vi "写入excel(幅频响应).vi"(7 "设置":string[](array[string])=["160", "10", "0.02", "0.02", "0.1", "10", "J5", "J6"], 8 "error in (no error)":errorcluster, 9 "被测幅值":dbl format="%.2p", 10 "参考幅值":dbl format="%.2p", 11 "NI_report输入":refnum<class "NI_report.lvclass">) -> (0 "error out":errorcluster, 3 "report out":refnum<class "NI_report.lvclass">)   [LabVIEW 2015]
uses:
  <vilib>/Utility/NIReport.llb/NI_report.lvclass
  <vilib>/addons/_office/_exclsub.llb/font.ctl
  Global.vi
  <vilib>/Utility/NIReport.llb/Excel/NI_Excel.lvclass
  <vilib>/addons/_office/NI_ReportGenerationToolkit.lvlib
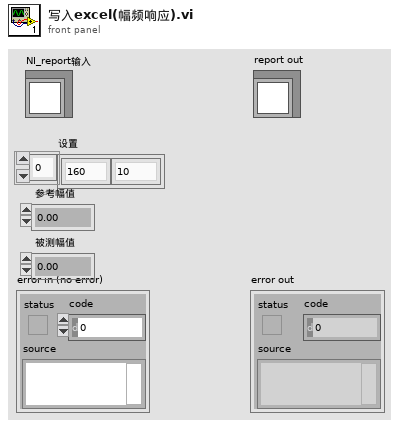
[diagram p1: front panel]
types:
  T1 = typedef "NI_ReportGenerationToolkit.lvlib/font.ctl" = cluster{"font name":string, "font size":dbl, "bold":u16, "italic":u16, "underline":u16, "strike through":u16, "font color":u32}
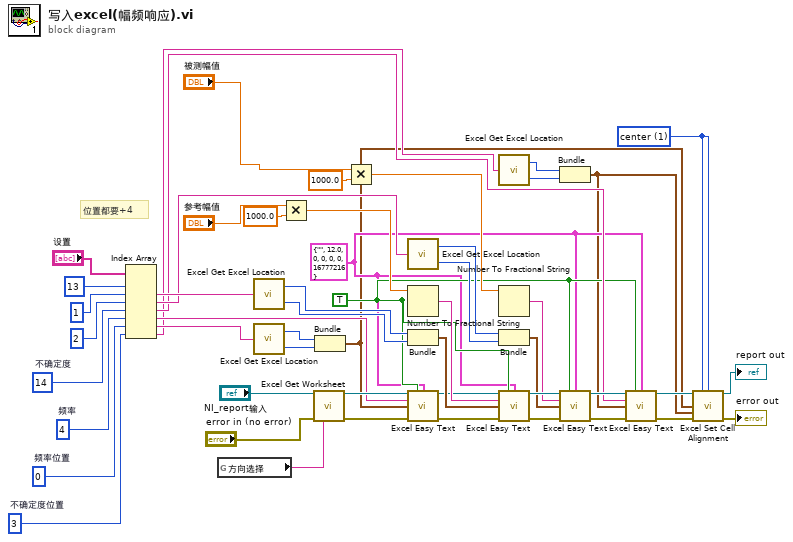
[diagram p0: block diagram]
diagram:
  w9 = 3  # 不确定度位置
  w23 = 0  # 频率位置
  w24 = 4  # 频率
  w25 = 14  # 不确定度
  w31 = 1 items=["top", "center", "bottom"] ("vertical alignment (top)")
  w5 = TRUE ("border? (F)")
  w4 = T1 {"font name"="", "font size"=12.0, "bold"=0, "italic"=0, "underline"=0, "strike through"=0, "font color"=16777216} ("font")
  # "位置都要+4"
  n1 = Index Array(array="设置", index #1=13 ("索引"), index #2=1 ("索引 (行)"), index #3=2 ("索引"), index #4=w25, index #5=w24, index #6=w23, index #7=w9) -> (element #2=w44:string, element #3=w38:string, element #4=w10:string, element #5=w20:string, element #6=w19:string, element #7=w8:string)  [unwired: 1 out]
  n2 = global read "Global.vi" "方向选择"() -> (w50:string)
  n3 = call <vilib>:"Excel Get Excel Location.vi"("cell's name"=w44) -> ("row"=w43:i32, "column"=w42:i32)
  n4 = call <vilib>:"Excel Get Excel Location.vi"("cell's name"=w19) -> ("row"=w18:i32, "column"=w17:i32)
  n5 = Multiply(x="参考幅值", y=1000.0) -> (x*y=w26:dbl)
  n6 = call <vilib>:"Excel Get Worksheet.vi"("report in"="NI_report输入", "error in (no error)"="error in (no error)", "name (\"\")"=w50) -> ("report out"=w22:refnum<class "NI_report.lvclass">, "error out"=w21:errorcluster)  [unwired: 11 in]
  n7 = Bundle("row"=w18, "column"=w17) -> (w3:cluster{"row":i32, "column":i32})  [unwired: 1 in]
  n8 = Multiply(x="被测幅值", y=1000.0) -> (x*y=w29:dbl)
  n9 = call <vilib>:"Excel Get Excel Location.vi"("cell's name"=w38) -> ("row"=w37:i32, "column"=w36:i32)
  n10 = Number To Fractional String(number=w26) -> (F-format string=w45:string)  [unwired: 3 in]
  n11 = Bundle("row"=w43, "column"=w42) -> (w33:cluster{"row":i32, "column":i32})  [unwired: 1 in]
  n12 = call <vilib>:"Excel Easy Text.vi"("report in"=w22, "border? (F)"=w5, "font"=w4, "text"=w20, "start (-1, -1)"=w3, "error in (no error)"=w21) -> ("report out"=w16:refnum<class "NI_report.lvclass">, "error out"=w15:errorcluster)  [unwired: 5 in, 3 out]
  n13 = call <vilib>:"Excel Get Excel Location.vi"("cell's name"=w8) -> ("row"=w7:i32, "column"=w6:i32)
  n14 = Number To Fractional String(number=w29) -> (F-format string=w39:string)  [unwired: 3 in]
  n15 = Bundle("row"=w37, "column"=w36) -> (w32:cluster{"row":i32, "column":i32})  [unwired: 1 in]
  n16 = call <vilib>:"Excel Easy Text.vi"("report in"=w16, "border? (F)"=w5, "font"=w4, "text"=w45, "start (-1, -1)"=w33, "error in (no error)"=w15) -> ("report out"=w41:refnum<class "NI_report.lvclass">, "error out"=w40:errorcluster)  [unwired: 5 in, 3 out]
  n17 = Bundle("row"=w7, "column"=w6) -> (w2:cluster{"row":i32, "column":i32})  [unwired: 1 in]
  n18 = call <vilib>:"Excel Easy Text.vi"("report in"=w41, "border? (F)"=w5, "font"=w4, "text"=w39, "start (-1, -1)"=w32, "error in (no error)"=w40) -> ("report out"=w14:refnum<class "NI_report.lvclass">, "error out"=w13:errorcluster)  [unwired: 5 in, 3 out]
  n19 = call <vilib>:"Excel Easy Text.vi"("report in"=w14, "border? (F)"=w5, "font"=w4, "text"=w10, "start (-1, -1)"=w2, "error in (no error)"=w13) -> ("report out"=w12:refnum<class "NI_report.lvclass">, "error out"=w11:errorcluster)  [unwired: 5 in, 3 out]
  n20 = call <vilib>:"Excel Set Cell Alignment.vi"("report in"=w12, "vertical alignment (top)"=w31, "horizontal alignment (left)"=w31, "start (-1, -1)"=w3, "end (-1, -1)"=w2, "error in (no error)"=w11) -> ("report out"=→"report out":refnum<class "NI_report.lvclass">, "error out"=→"error out":errorcluster)  [unwired: 8 in]
